vi "Create User Event - Stop.vi"(8 "error in (no error)":errorcluster) -> (0 "error out":errorcluster, 3 "User Event From MHL":refnum<user-event>)   [LabVIEW 2019, in "User Event - Stop.lvlib"]
doc: "Create a boolean user event that will be used to stop the event loop from the message handling loop."
uses:
  User Event - Stop.lvlib
  All User Events.ctl
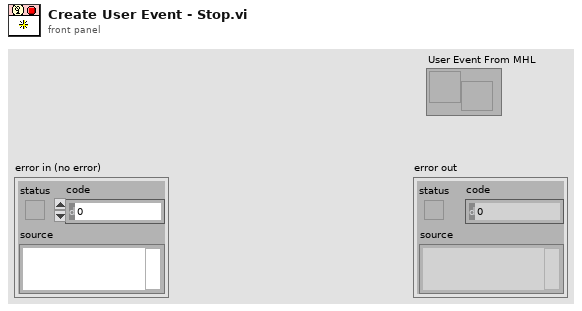
[diagram p1: front panel]
types:
  T1 = typedef "All User Events.ctl" = cluster{"User Event":string, "Event Data":variant}
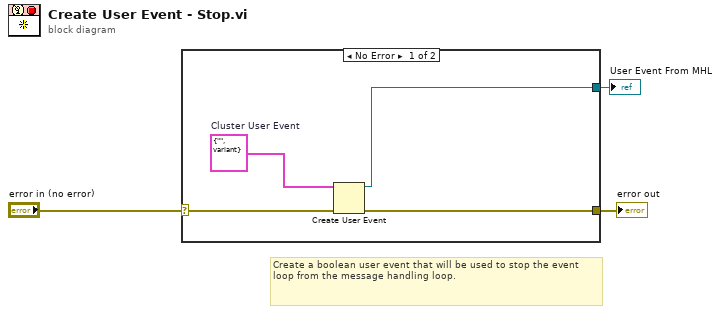
[diagram p0: block diagram]
diagram:
  # "Create a boolean user event that will be used to stop the event loop from the message handling loop."
  n1 = case shown="No Error" "error in (no error)" {
    selector: "error in (no error)" -> [w5 w8]
    tunnel: [w7 _] -> w1
    tunnel: [w6 w8] -> w3
    frame No Error {
      w4 = T1 {"User Event"="", "Event Data"=variant}  # Cluster User Event
      n2 = Create User Event(user event datatype=w4, error in=w5) -> (user event=w7:refnum<user-event>, error out=w6:errorcluster)
    }
    frame Error {
    }
  }
  "error out" <- w3
  "User Event From MHL" <- w1
